vi "Set to Delimited String.vi"(10 "delimiter":string=",", 11 "set":set{string}(c389)) -> (3 "delimited string":string)   [LabVIEW 2020, in "MeasurementLink Session Management.lvlib" / "Connection Map.lvclass"]
uses:
  Connection Map.lvclass
  Connection Map.lvclass/Connection Map.ctl
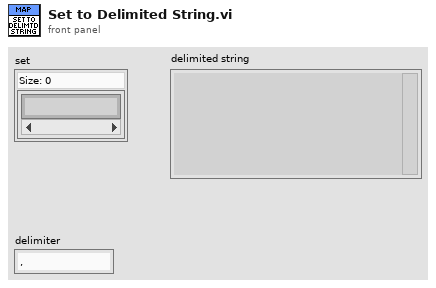
[diagram p1: front panel]
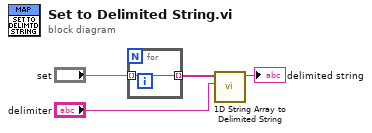
[diagram p0: block diagram]
diagram:
  n1 = for {
    tunnel: "set" -> [w5] mode=indexing
    tunnel: [w5] -> w3 mode=indexing
  }
  n2 = call <vilib>:"1D String Array to Delimited String.vi"("delimiter"="delimiter", "string array"=w3) -> ("delimited string"=→"delimited string":string)  [unwired: 9 in]
